vi "MT Generate System Parameters.vi"   [LabVIEW 2020, in "niDMT.lvlib"]
doc: "Calculates parameters for use with modulation and demodulation VIs. Wire the <B>system parameters</B> cluster from this VI to the corresponding parameter of the appropriate demodulation or modulation VI."
uses:
  <vilib>/addons/Modulation/niDMT.lvlib
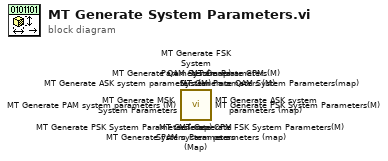
[diagram p0: block diagram]
diagram:
  n1 = call <vilib>:"MT Generate CPM System Parameters (Map).vi"() -> ()  [unwired: 14 in, 2 out]
  n2 = call <vilib>:"MT Generate CPM System Parameters (M).vi"() -> ()  [unwired: 13 in, 3 out]
  n3 = call <vilib>:"MT Generate MSK System Parameters.vi"() -> ()  [unwired: 13 in, 3 out]
  n4 = call <vilib>:"MT Generate ASK system parameters (map).vi"() -> ()  [unwired: 13 in, 3 out]
  n5 = call <vilib>:"MT Generate ASK system parameters (M).vi"() -> ()  [unwired: 13 in, 3 out]
  n6 = call <vilib>:"MT Generate FSK System Parameters(map).vi"() -> ()  [unwired: 13 in, 3 out]
  n7 = call <vilib>:"MT Generate FSK System Parameters(M).vi"() -> ()  [unwired: 13 in, 3 out]
  n8 = call <vilib>:"MT Generate PAM system parameters (M).vi"() -> ()  [unwired: 13 in, 3 out]
  n9 = call <vilib>:"MT Generate PAM system parameters (map).vi"() -> ()  [unwired: 13 in, 3 out]
  n10 = call <vilib>:"MT Generate PSK System Parameters(map).vi"() -> ()  [unwired: 13 in, 3 out]
  n11 = call <vilib>:"MT Generate PSK System Parameters(M).vi"() -> ()  [unwired: 13 in, 3 out]
  n12 = call <vilib>:"MT Generate QAM System Parameters(map).vi"() -> ()  [unwired: 13 in, 3 out]
  n13 = call <vilib>:"MT Generate QAM System Parameters(M).vi"() -> ()  [unwired: 13 in, 3 out]
